vi "Get First Child Item From Namespaced Element.vi"(8 "error in (no error)":errorcluster, 9 "Local Name":string, 10 "Namespace URI":string, 11 "DOM document in":refnum<k20>) -> (0 "error out":errorcluster, 2 "Value":string, 3 "DOM document out":refnum<k20>)   [LabVIEW 2012]
uses:
  <vilib>/xml/Close Reference(Node).vi
  <resource>/objmgr/DOMUserDefRef.rc
  <vilib>/xml/NI_XML.lvlib
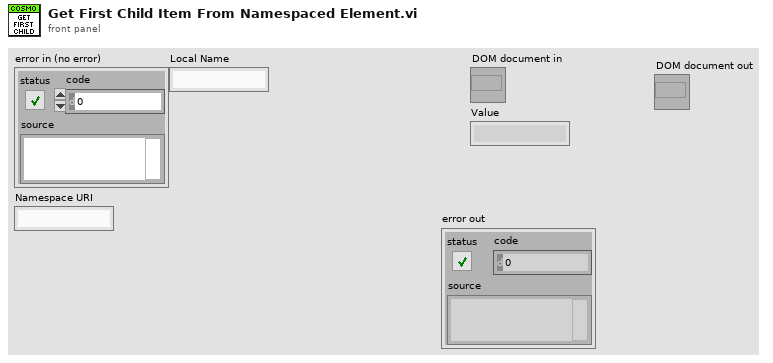
[diagram p1: front panel]
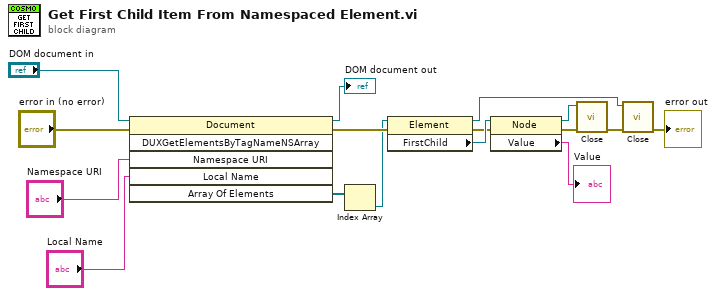
[diagram p0: block diagram]
diagram:
  n1 = invoke class="Document" method="DUXGetElementsByTagNameNSArray"(reference="DOM document in", error in="error in (no error)", "Namespace URI"="Namespace URI", "Local Name"="Local Name") -> (reference out=→"DOM document out":refnum<k20>, error out=w11:errorcluster, "Array Of Elements"=w2:refnum<k20>[])  [unwired: 2 in, 3 out]
  n2 = Index Array(array=w2) -> (element=w1:refnum<k20>)  [unwired: 1 in]
  n3 = property class="Element"(reference=w1, error in=w11) -> (reference out=w14:refnum<k20>, error out=w5:errorcluster, "FirstChild"=w6:refnum<k20>)
  n4 = property class="Node"(reference=w6, error in=w5) -> (reference out=w16:refnum<k20>, error out=w15:errorcluster, "Value"=→"Value":string)
  n5 = call-poly <vilib>:"Close.vi"("error in (no error)"=w15, "node"=w16) -> ("error out"=w3:errorcluster)  [unwired: 7 in]
  n6 = call-poly <vilib>:"Close.vi"("error in (no error)"=w3, "node"=w14) -> ("error out"=→"error out":errorcluster)  [unwired: 7 in]
